vi "Write Voltage Data to Optimization (Resync).vi"(5 "Network Data Array":T1[](array[typedef]), 7 "Bus by ID":T2[](array[typedef]), 8 "error in":errorcluster, 11 "Generic Optimization in":refnum<class "Generic Optimization.lvclass">) -> (0 "error out":errorcluster, 3 "Generic Optimization out":refnum<class "Generic Optimization.lvclass">)   [LabVIEW 2018, in "Resynchronization Actor.lvlib" / "Resynchronization.lvclass"]
uses:
  Resynchronization.lvclass
  Generic Optimization Actor/Generic Optimization/Generic Optimization.lvclass
  C:/Users/Administrator/Desktop/LabVIEW EMS/EMS Generic Actor/EMS Generic/EMS Generic.lvclass
  Generic Optimization Actor/Generic Optimization/Optimization Controls/Bus by ID.ctl
  <vilib>/ORNL/CSEISMIC DDS/CSEISMIC DDS Base/Data Types/Controls/DeviceID.ctl
  Generic Optimization Actor/Generic Optimization/Optimization Controls/Electrical Network Optimization Data.ctl
  <vilib>/ORNL/CSEISMIC DDS/CSEISMIC DDS Base/Data Types/SmartRelay_Measurement.ctl
  EMS Generic Actor/EMS Generic/EMS Generic.lvclass/EMS Generic.ctl
  Generic Optimization Actor/Generic Optimization/Optimization Controls/Bus Voltage.ctl
  <vilib>/ORNL/CSEISMIC DDS/CSEISMIC DDS Base/Data Types/DER_Measurement.ctl
  <vilib>/ORNL/CSEISMIC DDS/CSEISMIC DDS Base/Data Types/Meter_Measurement.ctl
  Global Variables/Global Variables.vi
  <vilib>/ORNL/CSEISMIC DDS/CSEISMIC DDS Base/CSEISMIC DDS.lvclass
  EMS Generic Actor/EMS Generic/EMS Generic.lvclass
  <vilib>/Analysis/NI_AALBase.lvlib
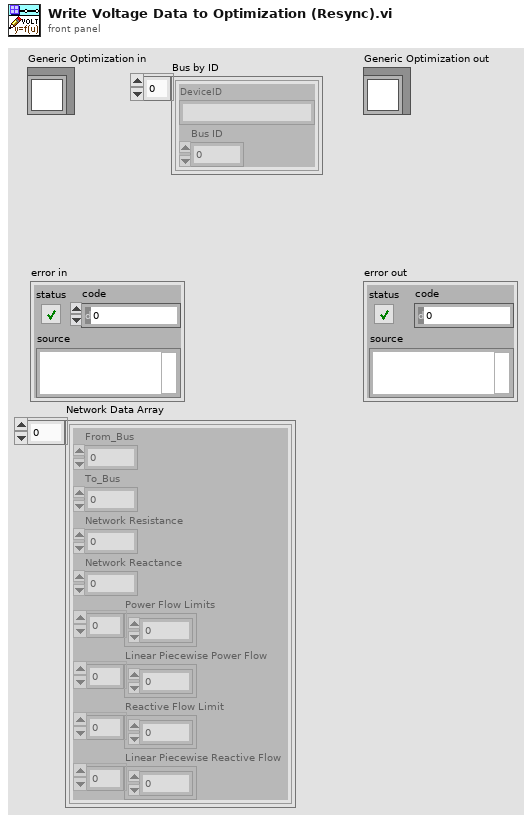
[diagram p1: front panel]
types:
  T1 = typedef "Generic Optimization Actor.lvlib/Generic Optimization.lvclass/Electrical Network Optimization Data.ctl" = cluster{"From_Bus":dbl, "To_Bus":dbl, "Network Resistance":dbl, "Network Reactance":dbl, "Power Flow Limits":dbl[], "Linear Piecewise Power Flow":dbl[], "Reactive Flow Limit":dbl[], "Linear Piecewise Reactive Flow":dbl[]}
  T2 = typedef "Generic Optimization Actor.lvlib/Generic Optimization.lvclass/Bus by ID.ctl" = cluster{"DeviceID":T3, "Bus ID":dbl}
  T3 = typedef "CSEISMIC DDS.lvlib/CSEISMIC DDS.lvclass/DeviceID.ctl" = string
  T4 = typedef "CSEISMIC DDS.lvlib/CSEISMIC DDS.lvclass/SmartRelay_Measurement.ctl" = cluster{"DeviceID":T3, "PrimaryVoltage":dbl[], "SecondaryVoltage":dbl[], "Current":dbl[], "RealPower":dbl[], "ReactivePower":dbl[], "LineConfig":u8[], "Frequency":dbl}
  T5 = typedef "Generic Optimization Actor.lvlib/Generic Optimization.lvclass/Bus Voltage.ctl" = cluster{"Bus":dbl, "Voltage":dbl}
  T6 = typedef "CSEISMIC DDS.lvlib/CSEISMIC DDS.lvclass/Meter_Measurement.ctl" = cluster{"DeviceID":T3, "Voltage":dbl[], "Current":dbl[], "RealPower":dbl[], "ReactivePower":dbl[], "LineConfig":u8[], "Frequency":dbl}
  T7 = typedef "CSEISMIC DDS.lvlib/CSEISMIC DDS.lvclass/DER_Measurement.ctl" = cluster{"DeviceID":T3, "Voltage":dbl[], "Current":dbl[], "RealPower":dbl[], "ReactivePower":dbl[], "LineConfig":u8[], "Frequency":dbl}
  T8 = typedef "EMS Generic Actor.lvlib/EMS Generic.lvclass/Data Type DVRs.ctl" = cluster{"IED_Status":refnum<data-value>, "IED_Status_0":refnum<data-value>, "DER_Measurement":refnum<data-value>, "DER_Info":refnum<data-value>, "DER_Status":refnum<data-value>, "ES_Measurement":refnum<data-value>, "ES_Info":refnum<data-value>, "PV_Info":refnum<data-value>, "SmartRelay_Info":refnum<data-value>, "SmartRelay_Measurement":refnum<data-value>, "Meter_Info":refnum<data-value>, "Meter_Measurement":refnum<data-value>, "HVAC_Status":refnum<data-value>, "HVAC_Measurement":refnum<data-value>, "PriceData_RealTime":refnum<data-value>, "PriceData_Demand":refnum<data-value>, "PriceData_Energy":refnum<data-value>, "ForecastData_Long":refnum<data-value>, "ForecastData_Short":refnum<data-value>, "DER_Control":refnum<data-value>, "DER_SetPointF":refnum<data-value>, "DER_SetPointP":refnum<data-value>, "DER_SetPointQ":refnum<data-value>, "DER_SetPointPF":refnum<data-value>, "DER_SetPointV":refnum<data-value>, "PV_setCurtailment":refnum<data-value>, "PV_setRampRate":refnum<data-value>, "Relay_Control":refnum<data-value>, "Load_Control":refnum<data-value>, "HVAC_Control":refnum<data-value>, "Generator_Info":refnum<data-value>, "ForecastData_Long_Backup":refnum<data-value>, "PriceData_RealTime_Backup":refnum<data-value>}
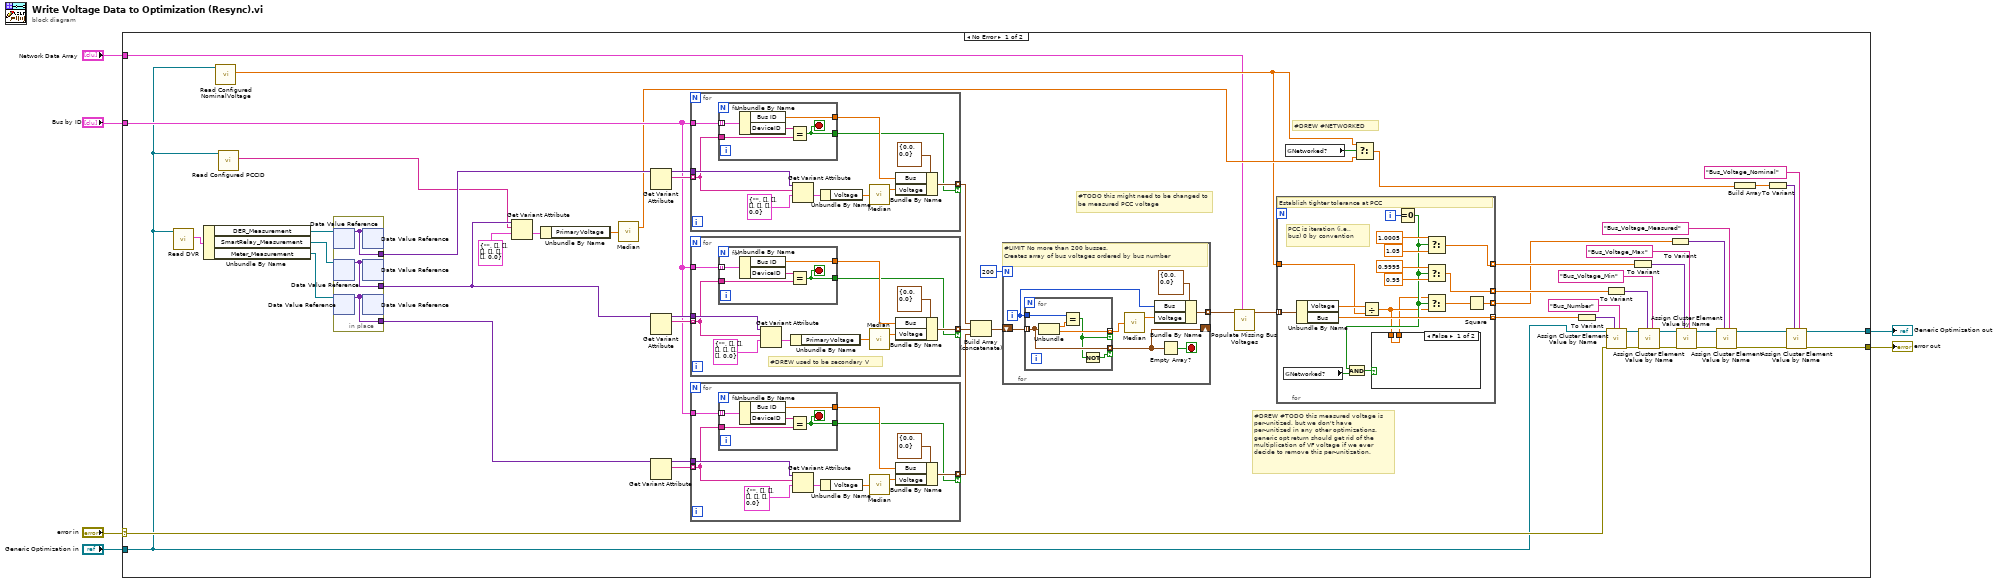
[diagram p0: block diagram]
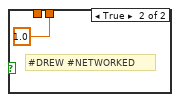
[diagram p2: hidden frame]
diagram:
  n1 = case shown="No Error" "error in" {
    selector: "error in" -> [w49 w150]
    tunnel: [w17 w150] -> w6
    tunnel: "Bus by ID" -> [w30 _]
    tunnel: "Generic Optimization in" -> [w8 w149]
    tunnel: [w7 w149] -> w2
    tunnel: "Network Data Array" -> [w9 _]
    frame No Error {
      # "#TODO this might need to be changed to be measured PCC voltage"
      # "#DREW #TODO this measured voltage is per-unitized, but we don't have per-unitized in any other optimizations.  generic opt return should get rid of the multiplication of VF voltage if we ever decide to remove this per-unitization."
      # "#DREW #NETWORKED"
      n2 = call "Read DVR.vi"("EMS Generic in"=w8) -> ("DVR"=w44:T8)  [unwired: 9 in, 1 out]
      n3 = Unbundle By Name(w44) -> ("DER_Measurement"=w43:refnum<data-value>, "SmartRelay_Measurement"=w42:refnum<data-value>, "Meter_Measurement"=w29:refnum<data-value>)
      n4 = call "Read Configured NominalVoltage.vi"("EMS Generic in"=w8) -> ("NominalVoltage"=w12:dbl)  [unwired: 8 in, 2 out]
      n5 = call "Read Configured PCCID.vi"("EMS Generic in"=w8) -> ("PCCID"=w13:T3)  [unwired: 8 in, 2 out]
      n6 = in-place {
        in-place-border: [w148] -> w28
        in-place-border: [w147] -> w26
        in-place-border: [w146] -> w27
        n7 = in-place-dvr #1(w43) -> (w148:variant)  [unwired: 1 out]
        n8 = in-place-dvr #2(w42) -> (w147:variant)  [unwired: 1 out]
        n9 = in-place-dvr #3(w29) -> (w146:variant)  [unwired: 1 out]
        n10 = in-place-dvr #1(w148) -> ()  [unwired: 2 out]
        n11 = in-place-dvr #2(w147) -> ()  [unwired: 2 out]
        n12 = in-place-dvr #3(w146) -> ()  [unwired: 2 out]
      }
      n13 = Get Variant Attribute(Variant=w26, name=w13, default value (empty Variant)=T4 {"DeviceID"="", "PrimaryVoltage"=[], "SecondaryVoltage"=[], "Current"=[], "RealPower"=[], "ReactivePower"=[], "LineConfig"=[], "Frequency"=0.0} ("SmartRelay_Measurement")) -> (value=w24:T4)  [unwired: 1 in, 3 out]
      n14 = Unbundle By Name(w24) -> ("PrimaryVoltage"=w23:dbl[])
      n15 = call <vilib>:"Median.vi"("X"=w23) -> ("median"=w14:dbl)  [unwired: 1 out]
      n16 = Get Variant Attribute(Variant=w28) -> (duplicate Variant=w40:variant, names=w41:string[])  [unwired: 3 in, 2 out]
      n17 = Get Variant Attribute(Variant=w26) -> (duplicate Variant=w39:variant, names=w38:string[])  [unwired: 3 in, 2 out]
      n18 = Get Variant Attribute(Variant=w27) -> (duplicate Variant=w36:variant, names=w37:string[])  [unwired: 3 in, 2 out]
      n19 = for {
        tunnel: w41 -> [w138] mode=indexing
        tunnel: w40 -> [w140]
        tunnel: w30 -> [w139]
        tunnel: [w136] -> w35 mode=indexing if=w130
        n20 = for {
          tunnel: w139 -> [w145] mode=indexing
          tunnel: w138 -> [w144]
          tunnel: [w142] -> w132
          tunnel: [w141] -> w130
          stop <- w141 stop-if-true
          n21 = Unbundle By Name(w145) -> ("Bus ID"=w142:dbl, "DeviceID"=w143:T3)
          n22 = Equal?(x=w143, y=w144) -> (x = y?=w141:bool)
        }
        n23 = Get Variant Attribute(Variant=w140, name=w138, default value (empty Variant)=T7 {"DeviceID"="", "Voltage"=[], "Current"=[], "RealPower"=[], "ReactivePower"=[], "LineConfig"=[], "Frequency"=0.0} ("DER_Measurement")) -> (value=w137:T7)  [unwired: 1 in, 3 out]
        n24 = Unbundle By Name(w137) -> ("Voltage"=w134:dbl[])
        n25 = call <vilib>:"Median.vi"("X"=w134) -> ("median"=w133:dbl)  [unwired: 1 out]
        n26 = Bundle By Name(cluster=T5 {"Bus"=0.0, "Voltage"=0.0} ("Bus Voltage"), "Bus"=w132, "Voltage"=w133) -> (w136:T5)
      }
      n27 = for {
        tunnel: w38 -> [w122] mode=indexing
        tunnel: w39 -> [w124]
        tunnel: w30 -> [w123]
        tunnel: [w120] -> w34 mode=indexing if=w115
        # "#DREW used to be secondary V"
        n28 = for {
          tunnel: w123 -> [w129] mode=indexing
          tunnel: w122 -> [w128]
          tunnel: [w126] -> w117
          tunnel: [w125] -> w115
          stop <- w125 stop-if-true
          n29 = Unbundle By Name(w129) -> ("Bus ID"=w126:dbl, "DeviceID"=w127:T3)
          n30 = Equal?(x=w127, y=w128) -> (x = y?=w125:bool)
        }
        n31 = Get Variant Attribute(Variant=w124, name=w122, default value (empty Variant)=T4 {"DeviceID"="", "PrimaryVoltage"=[], "SecondaryVoltage"=[], "Current"=[], "RealPower"=[], "ReactivePower"=[], "LineConfig"=[], "Frequency"=0.0} ("SmartRelay_Measurement")) -> (value=w121:T4)  [unwired: 1 in, 3 out]
        n32 = Unbundle By Name(w121) -> ("PrimaryVoltage"=w119:dbl[])
        n33 = call <vilib>:"Median.vi"("X"=w119) -> ("median"=w118:dbl)  [unwired: 1 out]
        n34 = Bundle By Name(cluster=T5 {"Bus"=0.0, "Voltage"=0.0} ("Bus Voltage"), "Bus"=w117, "Voltage"=w118) -> (w120:T5)
      }
      n35 = for {
        tunnel: w37 -> [w106] mode=indexing
        tunnel: w36 -> [w108]
        tunnel: w30 -> [w107]
        tunnel: [w104] -> w33 mode=indexing if=w99
        n36 = for {
          tunnel: w107 -> [w113] mode=indexing
          tunnel: w106 -> [w112]
          tunnel: [w110] -> w101
          tunnel: [w109] -> w99
          stop <- w109 stop-if-true
          n37 = Unbundle By Name(w113) -> ("Bus ID"=w110:dbl, "DeviceID"=w111:T3)
          n38 = Equal?(x=w111, y=w112) -> (x = y?=w109:bool)
        }
        n39 = Get Variant Attribute(Variant=w108, name=w106, default value (empty Variant)=T6 {"DeviceID"="", "Voltage"=[], "Current"=[], "RealPower"=[], "ReactivePower"=[], "LineConfig"=[], "Frequency"=0.0} ("Meter_Measurement")) -> (value=w105:T6)  [unwired: 1 in, 3 out]
        n40 = Unbundle By Name(w105) -> ("Voltage"=w103:dbl[])
        n41 = call <vilib>:"Median.vi"("X"=w103) -> ("median"=w102:dbl)  [unwired: 1 out]
        n42 = Bundle By Name(cluster=T5 {"Bus"=0.0, "Voltage"=0.0} ("Bus Voltage"), "Bus"=w101, "Voltage"=w102) -> (w104:T5)
      }
      n43 = Build Array (concatenate)(w35, w34, w33) -> (w32:T5[])
      n44 = for {
        N: 200 -> [_]
        shift-right: [w90] -> _
        shift-left: w32 -> [w91]
        tunnel: [w84] -> w11 mode=indexing
        i -> [w86]
        stop <- w89 stop-if-true
        # "#LIMIT No more than 200 busses.\nCreates array of bus voltages ordered by bus number"
        n45 = for {
          tunnel: w91 -> [w94] mode=indexing
          tunnel: w86 -> [w97]
          tunnel: [w95] -> w88 mode=indexing if=w93
          tunnel: [w94] -> w90 mode=indexing if=w92
          n46 = Unbundle(w94) -> ("Bus"=w96:dbl, "Voltage"=w95:dbl)
          n47 = Equal?(x=w97, y=w96) -> (x = y?=w93:bool)
          n48 = Not(x=w93) -> (.not. x?=w92:bool)
        }
        n49 = call <vilib>:"Median.vi"("X"=w88) -> ("median"=w85:dbl)  [unwired: 1 out]
        n50 = Bundle By Name(cluster=T5 {"Bus"=0.0, "Voltage"=0.0} ("Bus Voltage"), "Bus"=w86, "Voltage"=w85) -> (w84:T5)
        n51 = Empty Array?(array=w90) -> (empty?=w89:bool)
      }
      n52 = call "Populate Missing Bus Voltages.vi"("Network Data Array"=w9, "Bus Voltage Array in"=w11) -> ("Bus Voltage Array out"=w10:T5[])  [unwired: 8 in, 1 out]
      n53 = for {
        tunnel: w10 -> [w81] mode=indexing
        tunnel: [w80] -> w45 mode=indexing
        tunnel: w12 -> [w69]
        tunnel: [w77] -> w46 mode=indexing
        tunnel: [w76] -> w47 mode=indexing
        tunnel: [w79] -> w48 mode=indexing
        i -> [w78]
        # "PCC is iteration (i.e., bus) 0 by convention"
        # "Establish tighter tolerance at PCC"
        n54 = global read "Global Variables.vi" "Networked?"() -> (w68:bool)
        n55 = Unbundle By Name(w81) -> ("Voltage"=w70:dbl, "Bus"=w79:dbl)
        n56 = Divide(x=w70, y=w69) -> (x/y=w65:dbl)
        n57 = Equal To 0?(x=w78) -> (x = 0?=w66:bool)
        n58 = And(x=w66, y=w68) -> (x .and. y?=w67:bool)
        n59 = case shown="False" w67 {
          tunnel: w65 -> [w82 _]
          tunnel: [w82 1.0] -> w64
          frame False {
          }
          frame True {
            # "#DREW #NETWORKED"
          }
        }
        n60 = Select(t=1.0005, s=w66, f=1.05) -> (s? t:f=w77:dbl)
        n61 = Select(t=0.9995, s=w66, f=0.95) -> (s? t:f=w76:dbl)
        n62 = Select(t=w64, s=w66, f=w65) -> (s? t:f=w75:dbl)
        n63 = Square(x=w75) -> (x^2=w80:dbl)
      }
      n64 = global read "Global Variables.vi" "Networked?"() -> (w16:bool)
      n65 = Select(t=w12, s=w16, f=w14) -> (s? t:f=w15:dbl)
      n66 = To Variant(anything=w48) -> (Variant=w50:variant)
      n67 = To Variant(anything=w47) -> (Variant=w52:variant)
      n68 = call "Assign Cluster Element Value by Name.vi"("Element Name"="Bus_Number" ("Keyword Name"), "Value"=w50, "error in"=w49, "Generic Optimization"=w8) -> ("error out"=w61:errorcluster, "Generic Optimization out"=w60:refnum<class "Generic Optimization.lvclass">)  [unwired: 6 in]
      n69 = To Variant(anything=w46) -> (Variant=w54:variant)
      n70 = call "Assign Cluster Element Value by Name.vi"("Element Name"="Bus_Voltage_Min" ("Keyword Name"), "Value"=w52, "error in"=w61, "Generic Optimization"=w60) -> ("error out"=w62:errorcluster, "Generic Optimization out"=w59:refnum<class "Generic Optimization.lvclass">)  [unwired: 6 in]
      n71 = To Variant(anything=w45) -> (Variant=w56:variant)
      n72 = call "Assign Cluster Element Value by Name.vi"("Element Name"="Bus_Voltage_Max" ("Keyword Name"), "Value"=w54, "error in"=w62, "Generic Optimization"=w59) -> ("error out"=w63:errorcluster, "Generic Optimization out"=w58:refnum<class "Generic Optimization.lvclass">)  [unwired: 6 in]
      n73 = call "Assign Cluster Element Value by Name.vi"("Element Name"="Bus_Voltage_Measured" ("Keyword Name"), "Value"=w56, "error in"=w63, "Generic Optimization"=w58) -> ("error out"=w18:errorcluster, "Generic Optimization out"=w19:refnum<class "Generic Optimization.lvclass">)  [unwired: 6 in]
      n74 = Build Array(w15) -> (w22:dbl[])
      n75 = To Variant(anything=w22) -> (Variant=w20:variant)
      n76 = call "Assign Cluster Element Value by Name.vi"("Element Name"="Bus_Voltage_Nominal" ("Keyword Name"), "Value"=w20, "error in"=w18, "Generic Optimization"=w19) -> ("error out"=w17:errorcluster, "Generic Optimization out"=w7:refnum<class "Generic Optimization.lvclass">)  [unwired: 6 in]
    }
    frame Error {
    }
  }
  "error out" <- w6
  "Generic Optimization out" <- w2
